vi "SLM_Norm_to1.vi"(3 "Array":cdb[][](array[numeric])) -> (1 "x/y":cdb[][](array[numeric]) format="%#_2g")   [LabVIEW 2024]
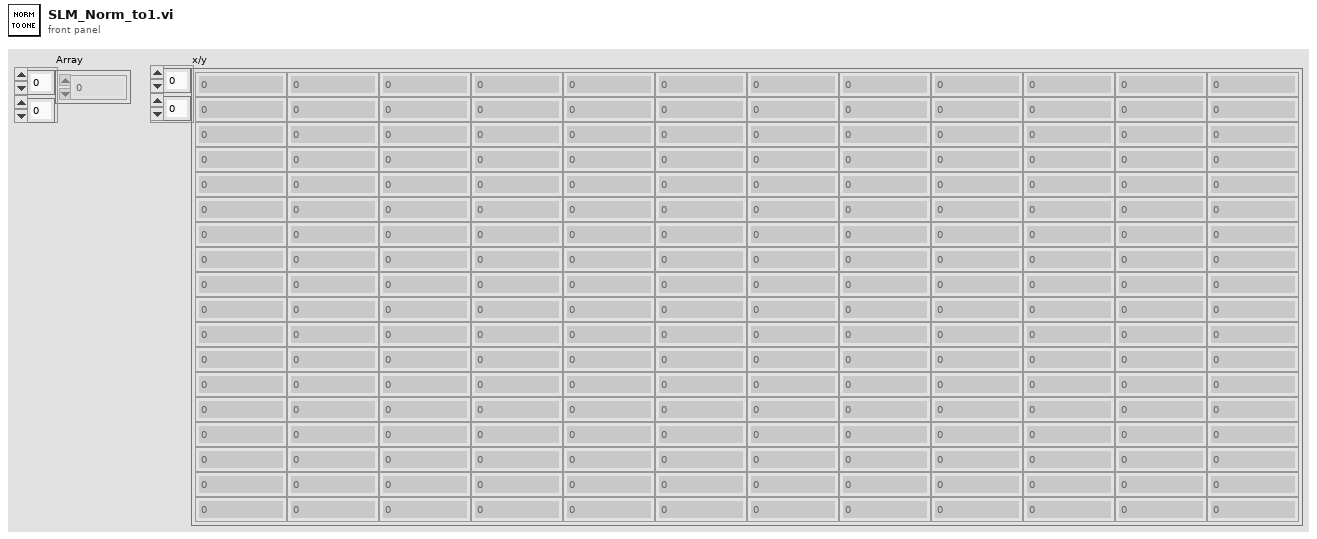
[diagram p1: front panel]
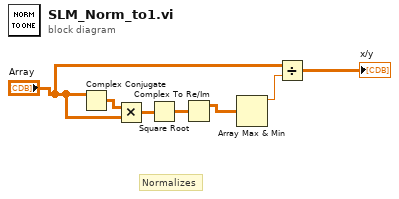
[diagram p0: block diagram]
diagram:
  # "Normalizes"
  n1 = Complex Conjugate(1:"Array") -> (0:w7:cdb[][])
  n2 = Multiply(x=w7, y="Array") -> (x*y=w6:cdb[][])
  n3 = Square Root(x=w6) -> (sqrt(x)=w5:cdb[][])
  n4 = Complex To Re/Im(x + iy=w5) -> (x=w4:dbl[][])  [unwired: 1 out]
  n5 = Array Max & Min(array=w4) -> (max value=w3:dbl)  [unwired: 3 out]
  n6 = Divide(x="Array", y=w3) -> (x/y=→"x/y":cdb[][])
